vi "Lissage de signal_base.vi"() -> ()   [LabVIEW 2018]
panel:
  in  "stop":bool
  out "Graphe déroulant":cluster{dbl, dbl, dbl}(graph)
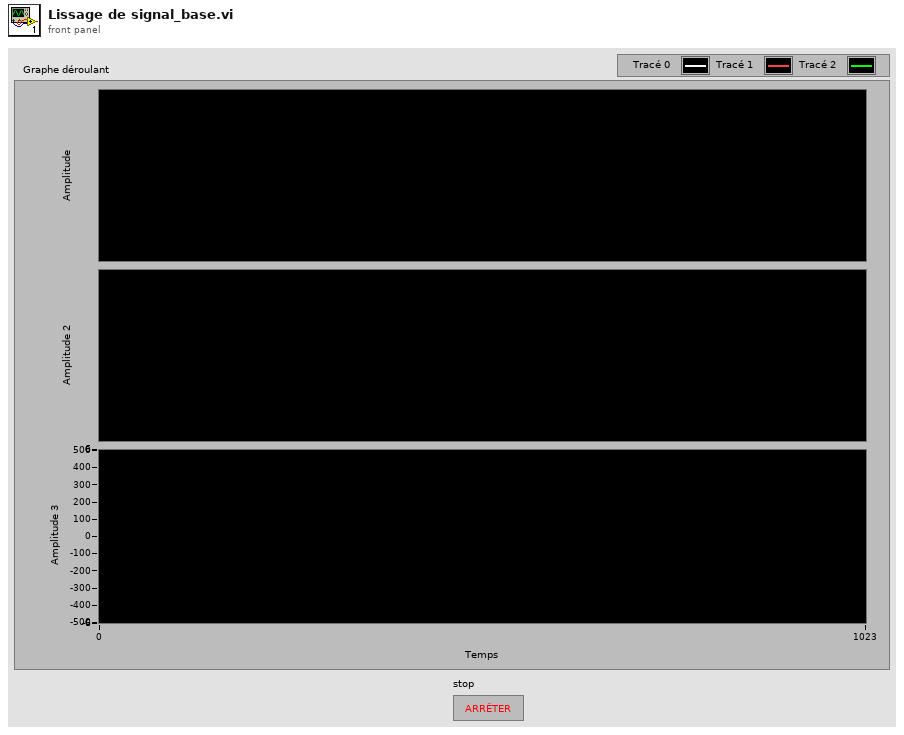
[diagram p1: front panel]
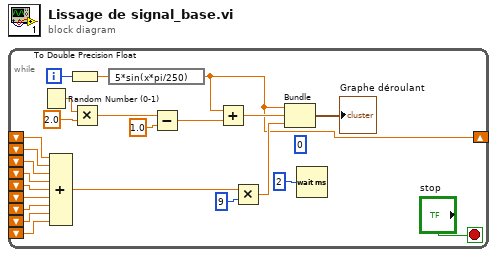
[diagram p0: block diagram]
diagram:
  n1 = while {
    shift-right: [w10] -> _
    shift-left: _ -> [w9]
    shift-left: _ -> [w8]
    shift-left: _ -> [w7]
    shift-left: _ -> [w6]
    shift-left: _ -> [w5]
    shift-left: _ -> [w4]
    shift-left: _ -> [w3]
    shift-left: _ -> [w2]
    shift-left: _ -> [w1]
    i -> [w21]
    stop <- "stop" stop-if-true
    (unwired) 0
    n2 = Random Number (0-1)() -> (number: 0 to 1=w19:dbl)
    n3 = Compound Arithmetic op=ADD(w9, w8, w7, w6, w5, w4, w3, w2, w1) -> (w13:dbl)
    n4 = To Double Precision Float(number=w21) -> (double precision float=w23:dbl)
    n5 = Multiply(x=w19, y=2.0) -> (x*y=w17:dbl)
    n6 = expression code="5*sin(x*pi/250)"(w23) -> (w10:dbl)
    n7 = Subtract(x=w17, y=1.0) -> (x-y=w16:dbl)
    n8 = Add(x=w10, y=w16) -> (x+y=w15:dbl)
    n9 = Multiply(x=w13, y=9) -> (x*y=w12:dbl)
    n10 = Bundle(w10, w15, w12) -> (→"Graphe déroulant":cluster{dbl, dbl, dbl})  [unwired: 1 in]
    n11 = Wait (ms)(milliseconds to wait=u32 2 ("attente (ms)")) -> ()  [unwired: 1 out]
  }
